vi "Check Elf In Range.vi"(10 "Grove":T2[][](array[typedef]), 11 "Elf Position":T1[](array[typedef])) -> (2 "Elf Present array":T2[](array[typedef]), 3 "Elf  in Range":bool)   [LabVIEW 2020]
uses:
  RB ENUM_Spot ID.ctl
  Cluster _Point Location.ctl
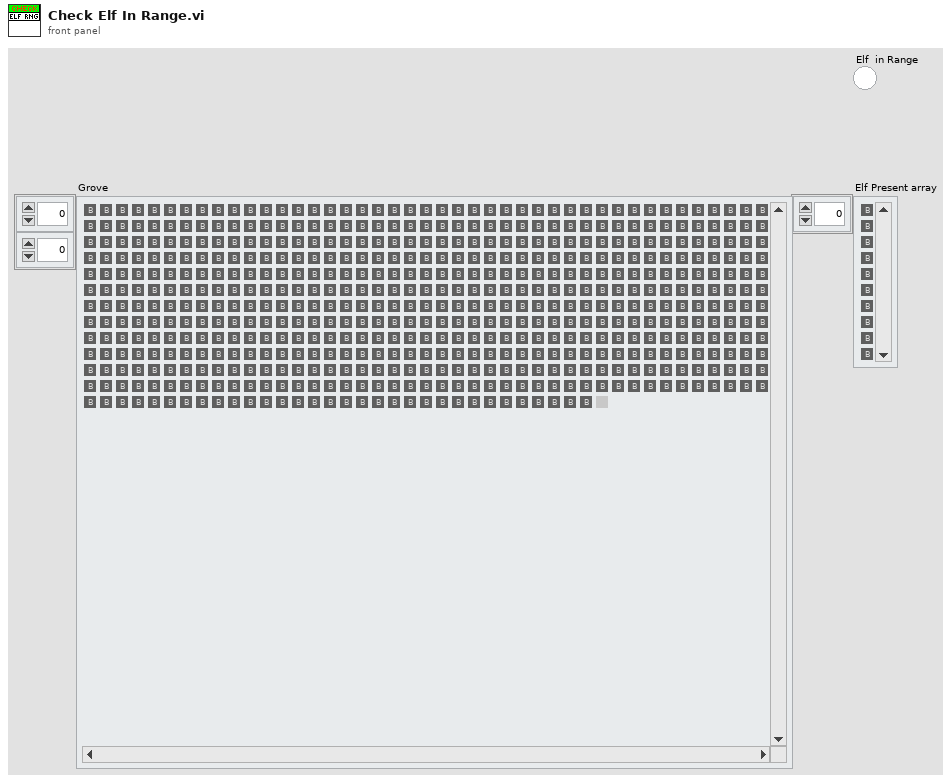
[diagram p1: front panel]
types:
  T1 = typedef "Cluster _Point Location.ctl" = cluster{"X col":i32, "Y row":i32}
  T2 = typedef "RB ENUM_Spot ID.ctl" = enum32{"Blank", "ELF", "Proposed"}
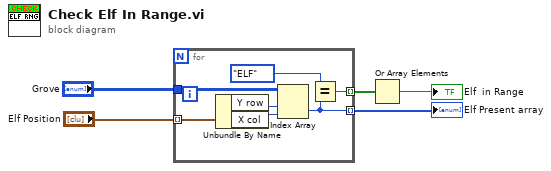
[diagram p0: block diagram]
diagram:
  n1 = for {
    tunnel: "Grove" -> [w12]
    tunnel: "Elf Position" -> [w11] mode=indexing
    tunnel: [w8] -> w5 mode=indexing
    tunnel: [w6] -> w2 mode=indexing
    n2 = Unbundle By Name(w11) -> ("Y row"=w10:i32, "X col"=w9:i32)
    n3 = Index Array(array=w12, index (row)=w10, index (col)=w9) -> (element=w8:T2)
    n4 = Equal?(x=RB_ENUM_Spot_ID."ELF" ("y"), y=w8) -> (x = y?=w6:bool)
  }
  "Elf Present array" <- w5
  n5 = Or Array Elements(Boolean array=w2) -> (logical OR=→"Elf  in Range":bool)
